vi "#163_MAV_MSG_AHRS.vi"(11 "mavlink_payload":u8[](array[numeric])) -> (3 "AHRS":T1)   [LabVIEW 2023]
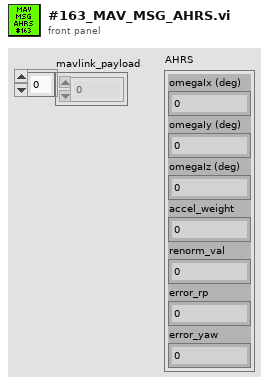
[diagram p1: front panel]
types:
  T1 = cluster{"omegaIx (deg)":sgl, "omegaIy (deg)":sgl, "omegaIz (deg)":sgl, "accel_weight":sgl, "renorm_val":sgl, "error_rp":sgl, "error_yaw":sgl}
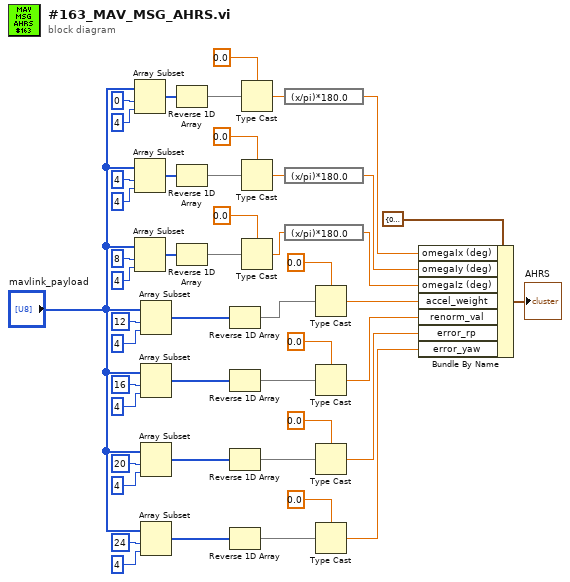
[diagram p0: block diagram]
diagram:
  n1 = Array Subset(array="mavlink_payload", index=0 ("Index"), length=4) -> (w47:u8[])
  n2 = Array Subset(array="mavlink_payload", index=4 ("Index"), length=4) -> (w38:u8[])
  n3 = Array Subset(array="mavlink_payload", index=8 ("Index"), length=4) -> (w32:u8[])
  n4 = Array Subset(array="mavlink_payload", index=12 ("Index"), length=4) -> (w24:u8[])
  n5 = Array Subset(array="mavlink_payload", index=16 ("Index"), length=4) -> (w18:u8[])
  n6 = Array Subset(array="mavlink_payload", index=20 ("Index"), length=4) -> (w12:u8[])
  n7 = Array Subset(array="mavlink_payload", index=24 ("Index"), length=4) -> (w6:u8[])
  n8 = Reverse 1D Array(array=w47) -> (reversed array=w46:u8[])
  n9 = Reverse 1D Array(array=w38) -> (reversed array=w37:u8[])
  n10 = Reverse 1D Array(array=w32) -> (reversed array=w31:u8[])
  n11 = Reverse 1D Array(array=w24) -> (reversed array=w23:u8[])
  n12 = Reverse 1D Array(array=w18) -> (reversed array=w17:u8[])
  n13 = Reverse 1D Array(array=w12) -> (reversed array=w11:u8[])
  n14 = Reverse 1D Array(array=w6) -> (reversed array=w5:u8[])
  n15 = Type Cast(type=sgl 0.0 ("Index"), x=w46) -> (*(type *) &x=w41:sgl)
  n16 = Type Cast(type=sgl 0.0 ("Index"), x=w37) -> (*(type *) &x=w34:sgl)
  n17 = Type Cast(type=sgl 0.0 ("Index"), x=w31) -> (*(type *) &x=w28:sgl)
  n18 = expression code="(x/pi)*180.0" ("radians to degrees")(w41) -> (w40:sgl)
  n19 = expression code="(x/pi)*180.0" ("radians to degrees")(w34) -> (w27:sgl)
  n20 = expression code="(x/pi)*180.0" ("radians to degrees")(w28) -> (w26:sgl)
  n21 = Type Cast(type=sgl 0.0 ("Index"), x=w23) -> (*(type *) &x=w20:sgl)
  n22 = Type Cast(type=sgl 0.0 ("Index"), x=w17) -> (*(type *) &x=w14:sgl)
  n23 = Type Cast(type=sgl 0.0 ("Index"), x=w11) -> (*(type *) &x=w8:sgl)
  n24 = Type Cast(type=sgl 0.0 ("Index"), x=w5) -> (*(type *) &x=w1:sgl)
  n25 = Bundle By Name(cluster=T1 {"omegaIx (deg)"=0.0, "omegaIy (deg)"=0.0, "omegaIz (deg)"=0.0, "accel_weight"=0.0, "renorm_val"=0.0, "error_rp"=0.0, "error_yaw"=0.0} ("AHRS"), "omegaIx (deg)"=w40, "omegaIy (deg)"=w27, "omegaIz (deg)"=w26, "accel_weight"=w20, "renorm_val"=w14, "error_rp"=w8, "error_yaw"=w1) -> (→"AHRS":T1)
